vi "ADIS16470 Loop.vi"(8 "error in":errorcluster) -> ()   [LabVIEW 2020]
uses:
  Typedef/ADIS16470 Device Reference.ctl
  Typedef/ADIS16470 Hardware Configuration.ctl
  <vilib>/Rock Robotics/WPI/SPI/WPI_SPIMode.ctl
  <vilib>/Rock Robotics/SystemInterfaces/DIO/FPGA_DIOChannel.ctl
  <vilib>/Rock Robotics/SystemInterfaces/spilib/spi_bus.ctl
  Typedef/ADIS16470 Status.ctl
  Typedef/ADIS16470 Data.ctl
  Typedef/ADIS16470 Process.ctl
  Typedef/ADIS16470 Command Type.ctl
  <vilib>/Rock Robotics/SystemInterfaces/CounterEncoderSourceConvertion/FPGA_CounterEncoderSourceConvertionLVSourceType.ctl
  <vilib>/Rock Robotics/SystemInterfaces/DIO/FPGA_DIODigitalSourceChannel.ctl
  <vilib>/Rock Robotics/SystemInterfaces/AnalogTrigger/FPGA_AnalogTriggerIndex.ctl
  <vilib>/Rock Robotics/SystemInterfaces/AnalogTrigger/FPGA_AnalogTriggerOutType.ctl
  <vilib>/Rock Robotics/WPI/SPI/WPI_SPIDevRef.ctl
  Typedef/ADIS16470 Register.ctl
  <vilib>/Rock Robotics/WPI/Counter/WPI_CounterDigitalInputToDigitalSource.vi
panel:
  out "Offset Bias":i16[](array[numeric])
  in  "ADIS16470DevRef":T1={"DevStatus"={"status"=FALSE, "code"=0, "source"=""}, "Hardware Config"={"SPI Clock Rate (Hz)"=1000000.0, "IMU SPI Mode (3)"=enum."Mode 3 (Clk Idle High,Sample on Trailing)", "IMU Reset Pin"=enum."SPI Port CS2", "IMU SPI Bus"=enum."SPI On-Board, CS0", "IMU Data Ready Pin"=enum."SPI Port CS1", "Stall Config"={"Pow2BytesPerRead"=255, "StallTicks"=640, "CsToSclkTicks"=5}}, "Calibration Complete"=refnum, "Status Reference"=refnum, "Position Reference"=refnum, "Velocity Reference"=refnum, "Sychronous Process VI"=refnum, "Cmd FIFO"=refnum, "Source"={"DevStatus"={"status"=FALSE, "code"=0, "source"=""}, "AnalogTriggerMode?"=FALSE, "DigitalMode"={"DIO Channel"=enum."Disabled"}, "AnalogTriggerMode"={"AnalogTriggerIndex"=enum."Trig 0", "OutputType"=enum."InWindow"}}, "Data FIFO"=refnum, "Calibration Time (ms)"=5}
  in  "Main Name":string
  # "XG_BIAS_LOW"
  # "XG_BIAS_HIGH"
  # "YG_BIAS_LOW"
  # "YG_BIAS_HIGH"
  # "ZG_BIAS_LOW"
  # "ZG_BIAS_HIGH"
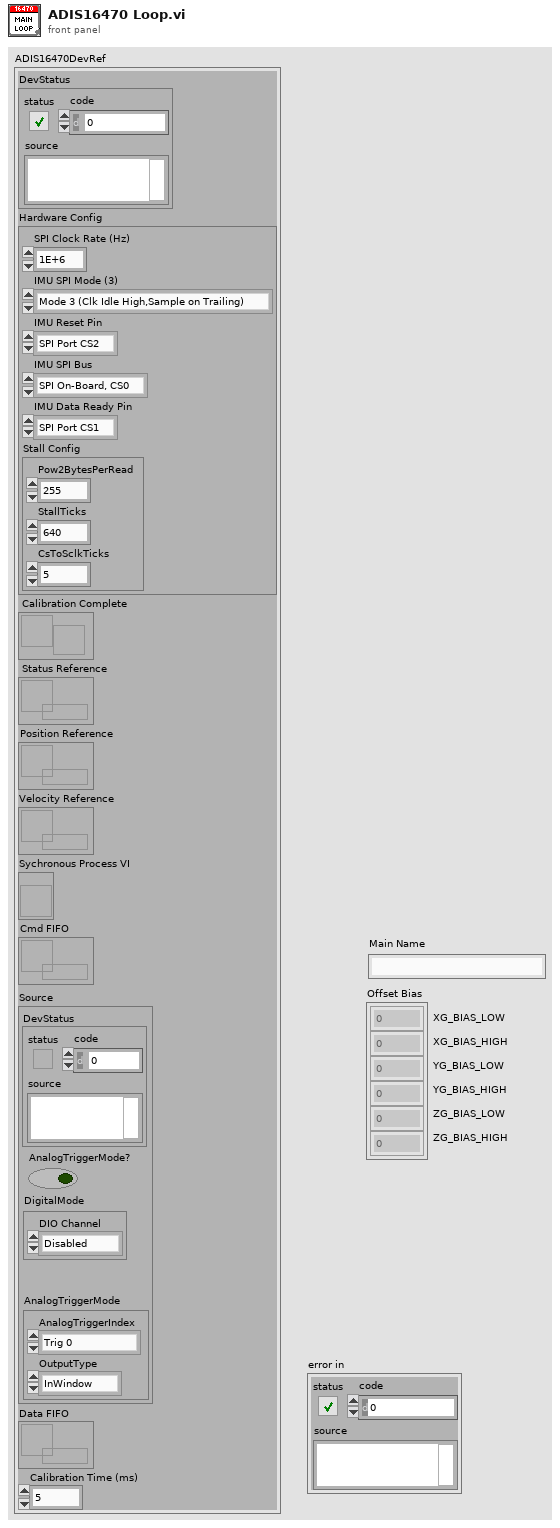
[diagram p1: front panel]
types:
  T1 = typedef "ADIS16470 Device Reference.ctl" = cluster{"DevStatus":errorcluster, "Hardware Config":T2, "Calibration Complete":refnum<notifier>, "Status Reference":refnum<data-value>, "Position Reference":refnum<data-value>, "Velocity Reference":refnum<data-value>, "Sychronous Process VI":T6, "Cmd FIFO":refnum<k33>, "Source":T7, "Data FIFO":refnum<k33>, "Calibration Time (ms)":u32}
  T2 = typedef "ADIS16470 Hardware Configuration.ctl" = cluster{"SPI Clock Rate (Hz)":dbl, "IMU SPI Mode (3)":T3, "IMU Reset Pin":T4, "IMU SPI Bus":T5, "IMU Data Ready Pin":T4, "Stall Config":cluster{"Pow2BytesPerRead":u8, "StallTicks":u16, "CsToSclkTicks":u8}}
  T3 = typedef "WPI_SPIMode.ctl" = enum16{"Mode 0 (Clk Idle Low,Sample on Leading)", "Mode 1 (Clk Idle Low,Sample on Trailing)", "Mode 2 (Clk Idle High,Sample on Leading)", "Mode 3 (Clk Idle High,Sample on Trailing)"}
  T4 = typedef "FPGA_DIOChannel.ctl" = enum8{"DIO 0", "DIO 1", "DIO 2", "DIO 3", "DIO 4", "DIO 5", "DIO 6", "DIO 7", "DIO 8", "DIO 9", "DIO MXP 0", "DIO MXP 1", "DIO MXP 2", "DIO MXP 3", "DIO MXP 4", "DIO MXP 5", "DIO MXP 6", "DIO MXP 7", "DIO MXP 8", "DIO MXP 9", "DIO MXP 10", "DIO MXP 11", "DIO MXP 12", "DIO MXP 13", "DIO MXP 14", "DIO MXP 15", "SPI Port CS1", "SPI Port CS2", "SPI Port CS3", "SPI Port MISO", "SPI Port MOSI", "Invalid"}
  T5 = typedef "spi_bus.ctl" = enum16{"SPI On-Board, CS0", "SPI On-Board, CS1", "SPI On-Board, CS2", "SPI On-Board, CS3", "SPI MXP", "Invalid"}
  T6 = typedef "ADIS16470 Process.ctl" = refnum<vi>
  T7 = typedef "FPGA_CounterEncoderSourceConvertionLVSourceType.ctl" = cluster{"DevStatus":errorcluster, "AnalogTriggerMode?":bool, "DigitalMode":cluster{"DIO Channel":T8}, "AnalogTriggerMode":cluster{"AnalogTriggerIndex":T9, "OutputType":T10}}
  T8 = typedef "FPGA_DIODigitalSourceChannel.ctl" = enum8{"DIO 0", "DIO 1", "DIO 2", "DIO 3", "DIO 4", "DIO 5", "DIO 6", "DIO 7", "DIO 8", "DIO 9", "DIO MXP 0", "DIO MXP 1", "DIO MXP 2", "DIO MXP 3", "DIO MXP 4", "DIO MXP 5", "DIO MXP 6", "DIO MXP 7", "DIO MXP 8", "DIO MXP 9", "DIO MXP 10", "DIO MXP 11", "DIO MXP 12", "DIO MXP 13", "DIO MXP 14", "DIO MXP 15", "SPI Port CS1", "SPI Port CS2", "SPI Port CS3", "SPI Port MISO", "SPI Port MOSI", "Disabled"}
  T9 = typedef "FPGA_AnalogTriggerIndex.ctl" = enum8{"Trig 0", "Trig 1", "Trig 2", "Trig 3", "Trig 4", "Trig 5", "Trig 6", "Trig 7", "Invalid"}
  T10 = typedef "FPGA_AnalogTriggerOutType.ctl" = enum16{"InWindow", "TriggerState", "Rising", "Falling"}
  T11 = typedef "WPI_SPIDevRef.ctl" = cluster{"DevStatus":errorcluster, "Handle":i32, "SPI Bus":T5}
  T12 = typedef "ADIS16470 Data.ctl" = cluster{"XAngle":dbl, "YAngle":dbl, "ZAngle":dbl}
  T13 = typedef "ADIS16470 Register.ctl" = u8
  T14 = cluster{"SPIDevRef":T11, "Data Counter":u16, "Reset":bool, "Digital Source":T7, "Bytes Per Sample":u32, "Position":T12, "Velocity":T12, "ADIS16470DevRef":T1, "TimeStampPrev":u32, "Sensor to Robot Rotation":dbl[][], "Data Packet":T13[], "AutoSPI Active?":bool, "Delay Factor":dbl}
  T15 = typedef "ADIS16470 Status.ctl" = cluster{"Calibrated?":bool, "IMU Detected?":bool}
  T16 = typedef "ADIS16470 Command Type.ctl" = cluster{"Command":enum16{"None", "Reset", "Recalibrate"}, "Data":u32}
  T17 = typedef "WPI_DigitalOutputDevRef.ctl" = cluster{"DIO Channel":T4, "DevStatus":errorcluster}
  T18 = typedef "WPI_DigitalInputDevRef.ctl" = cluster{"DevStatus":errorcluster, "DIO Channel":T4}
  T19 = cluster{"Pow2BytesPerRead":u8, "StallTicks":u16, "CsToSclkTicks":u8}
  T20 = enum32{"Bad", "Idle", "Run top level", "Running"}
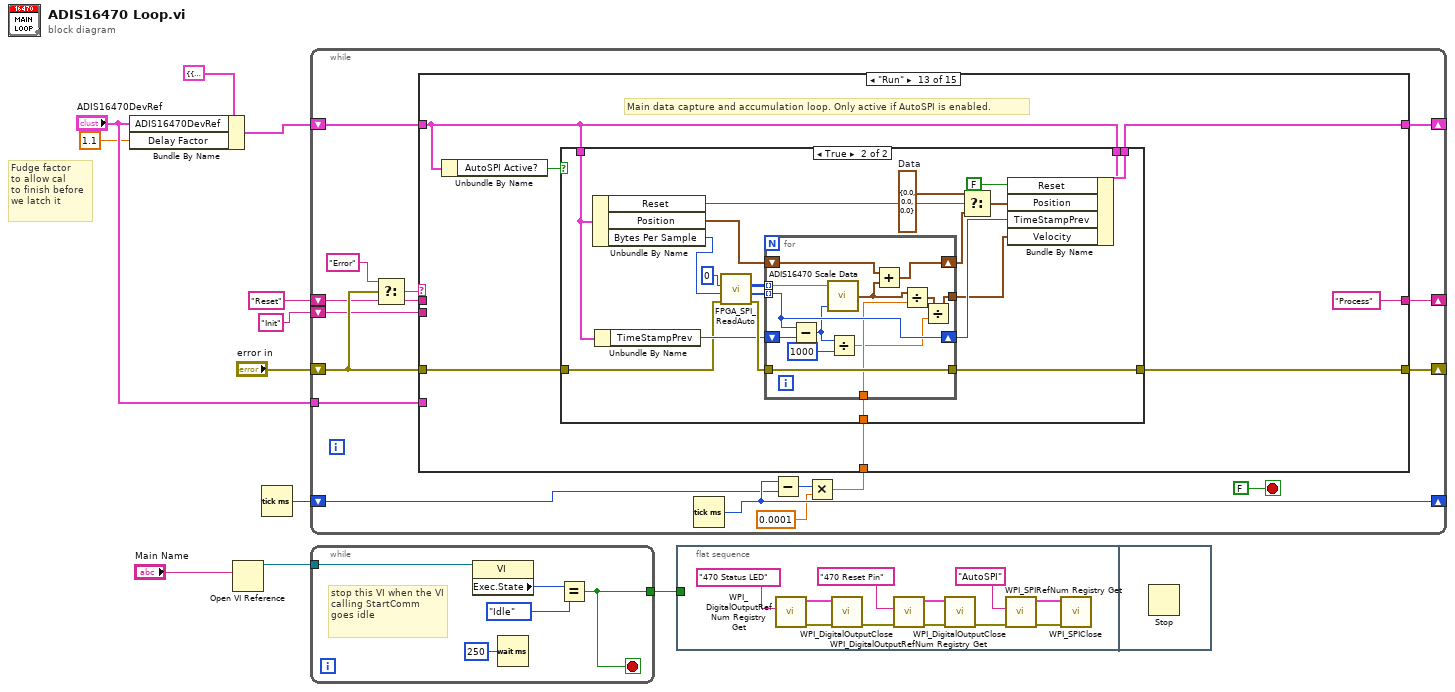
[diagram p0: block diagram]
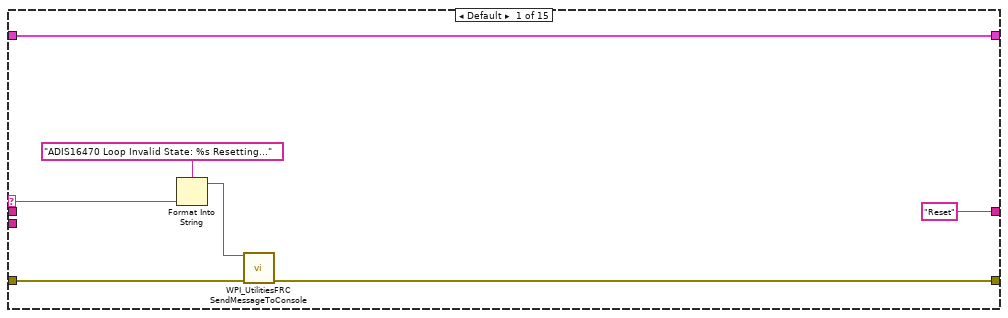
[diagram p2: hidden frame]
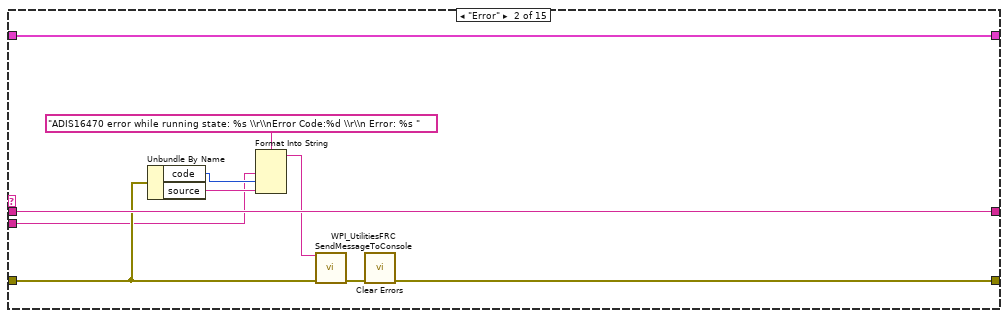
[diagram p3: hidden frame]
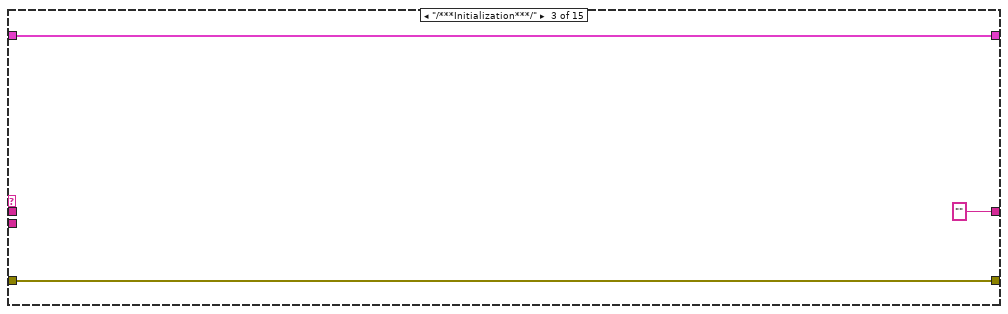
[diagram p4: hidden frame]
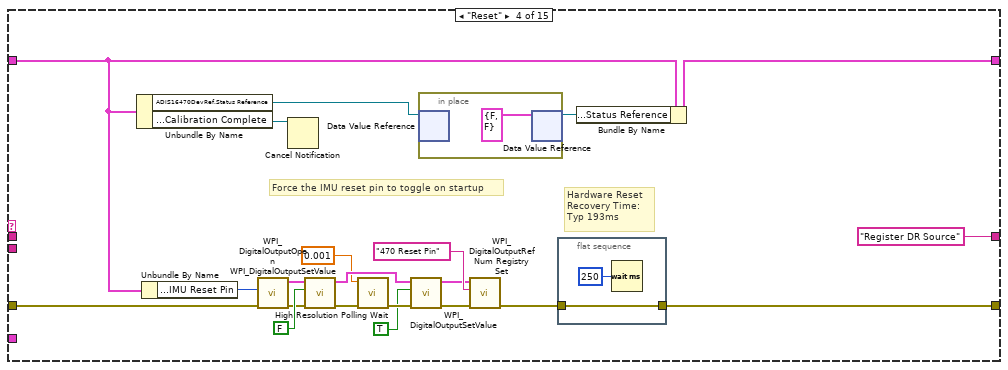
[diagram p5: hidden frame]
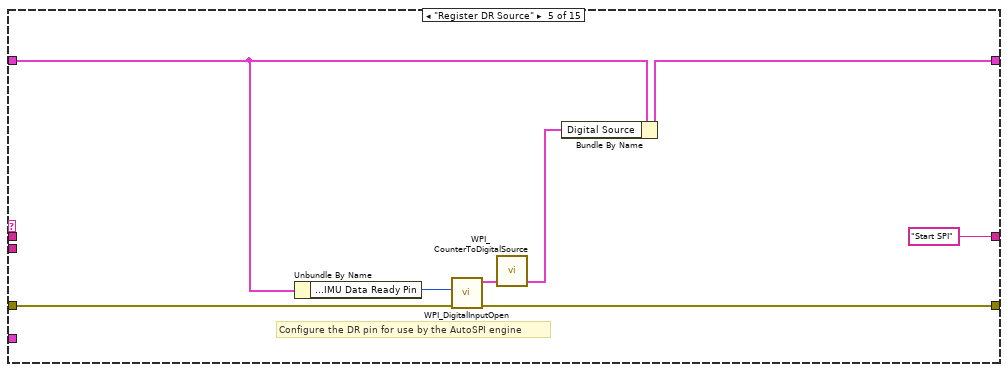
[diagram p6: hidden frame]
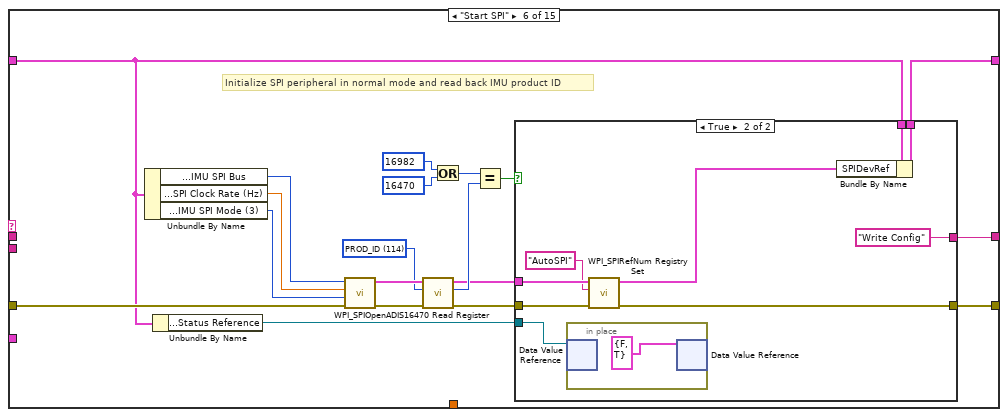
[diagram p7: hidden frame]
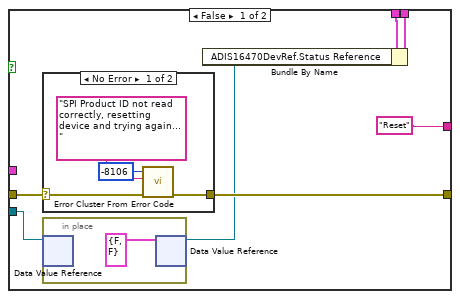
[diagram p8: hidden frame]
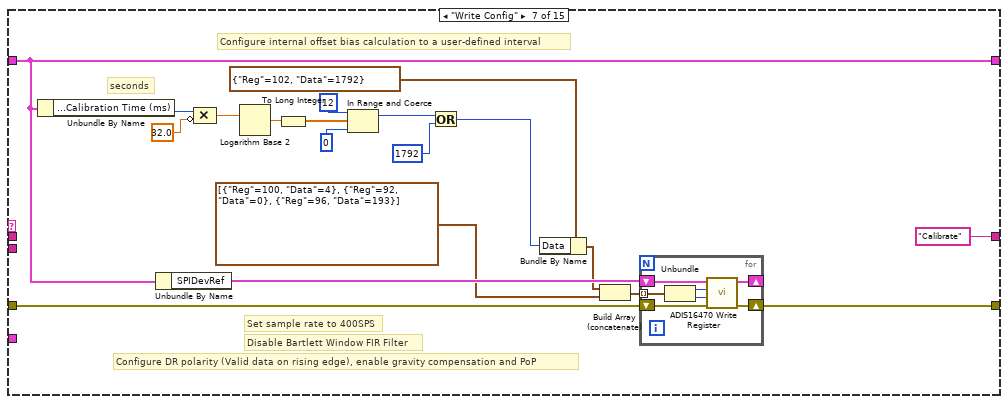
[diagram p10: hidden frame]
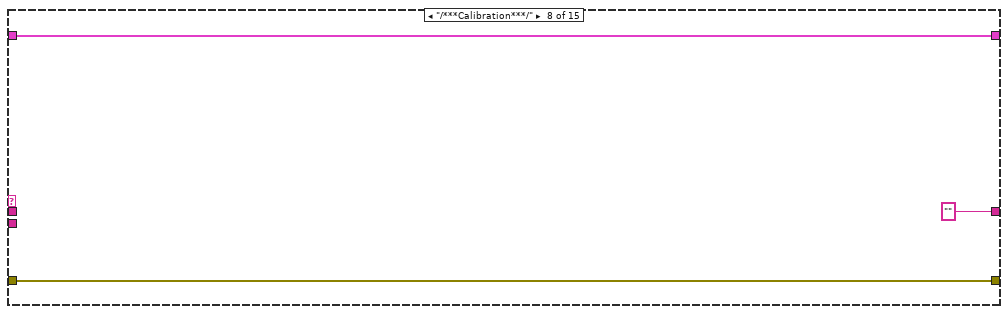
[diagram p11: hidden frame]
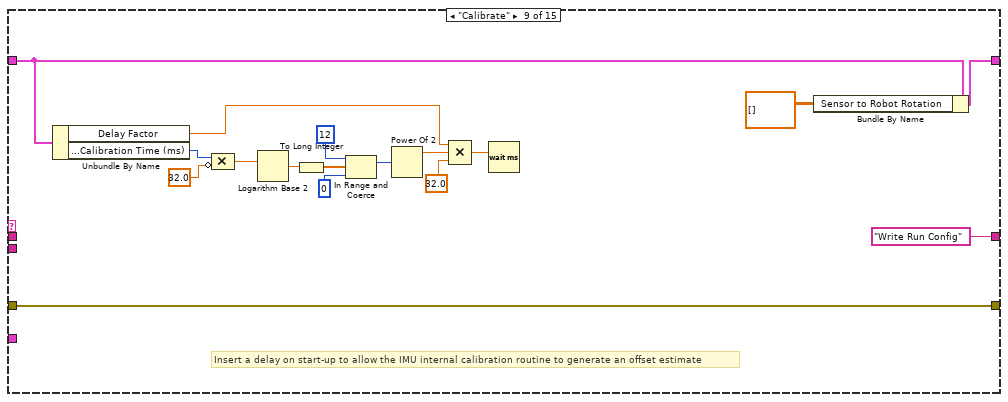
[diagram p12: hidden frame]
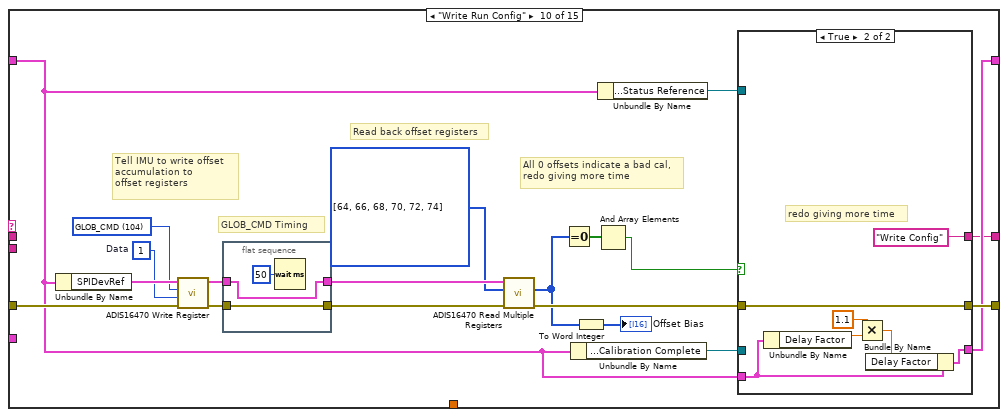
[diagram p13: hidden frame]
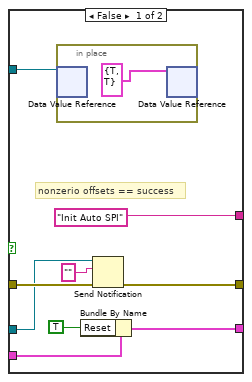
[diagram p14: hidden frame]
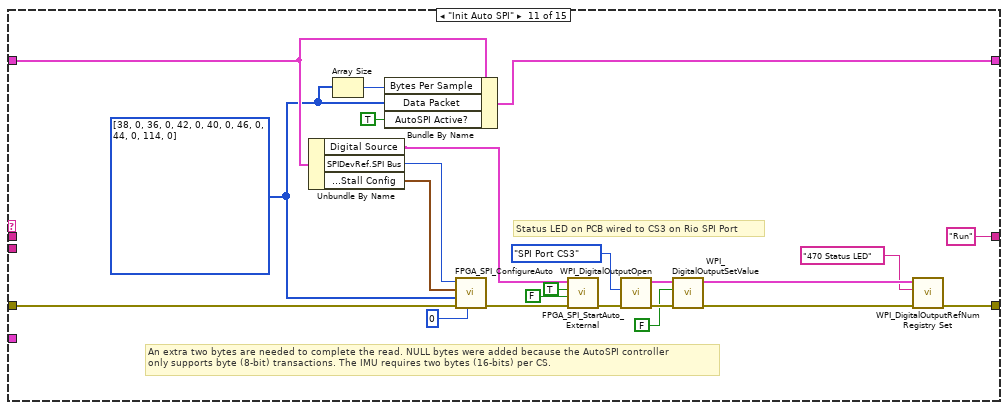
[diagram p15: hidden frame]
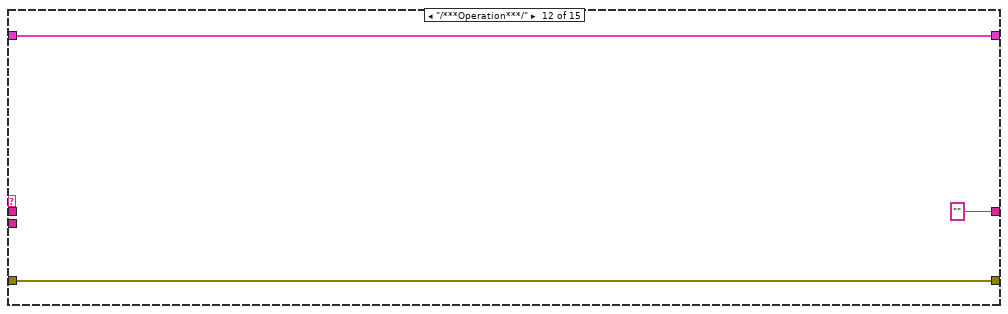
[diagram p16: hidden frame]
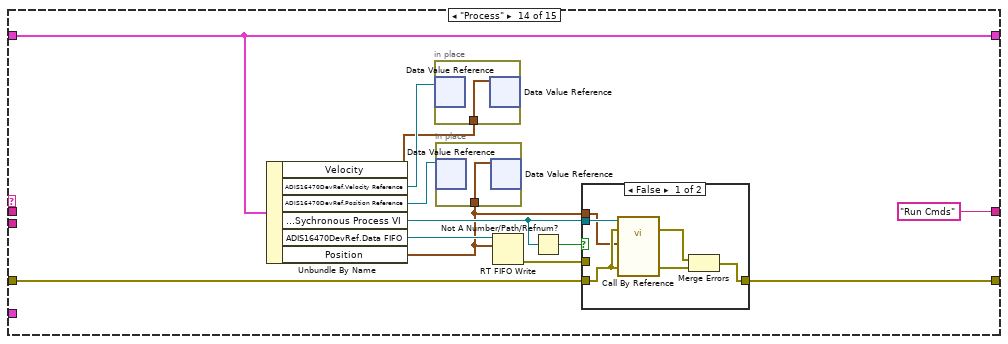
[diagram p18: hidden frame]
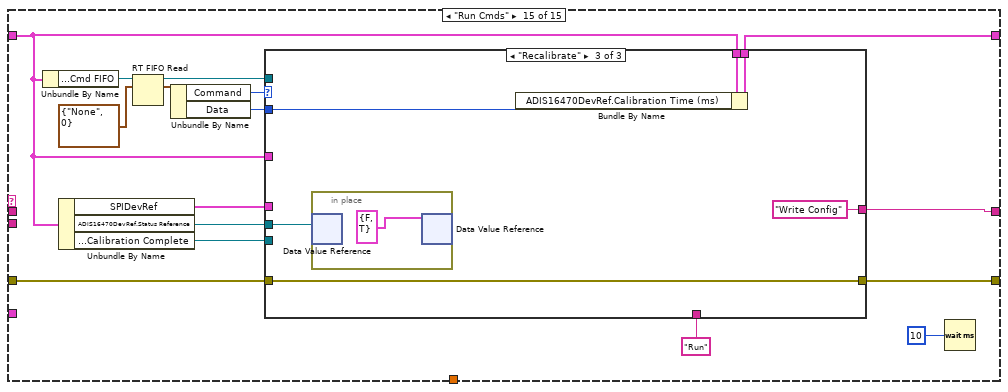
[diagram p20: hidden frame]
diagram:
  # "Fudge factor\nto allow cal\nto finish before\nwe latch it"
  n1 = Bundle By Name(cluster=T14 {"SPIDevRef"={"DevStatus"={"status"=FALSE, "code"=0, "source"=""}, "Handle"=0, "SPI Bus"=enum."SPI On-Board, CS0"}, "Data Counter"=0, "Reset"=FALSE, "Digital Source"={"DevStatus"={"status"=FALSE, "code"=0, "source"=""}, "AnalogTriggerMode?"=FALSE, "DigitalMode"={"DIO Channel"=enum."DIO 1"}, "AnalogTriggerMode"={"AnalogTriggerIndex"=enum."Trig 0", "OutputType"=enum."InWindow"}}, "Bytes Per Sample"=0, "Position"={"XAngle"=0.0, "YAngle"=0.0, "ZAngle"=0.0}, "Velocity"={"XAngle"=0.0, "YAngle"=0.0, "ZAngle"=0.0}, "ADIS16470DevRef"={"DevStatus"={"status"=FALSE, "code"=0, "source"=""}, "Hardware Config"={"SPI Clock Rate (Hz)"=1000000.0, "IMU SPI Mode (3)"=enum."Mode 3 (Clk Idle High,Sample on Trailing)", "IMU Reset Pin"=enum."SPI Port CS2", "IMU SPI Bus"=enum."SPI On-Board, CS0", "IMU Data Ready Pin"=enum."SPI Port CS1", "Stall Config"={"Pow2BytesPerRead"=255, "StallTicks"=640, "CsToSclkTicks"=5}}, "Calibration Complete"=refnum, "Status Reference"=refnum, "Position Reference"=refnum, "Velocity Reference"=refnum, "Sychronous Process VI"=refnum, "Cmd FIFO"=refnum, "Source"={"DevStatus"={"status"=FALSE, "code"=0, "source"=""}, "AnalogTriggerMode?"=FALSE, "DigitalMode"={"DIO Channel"=enum."Disabled"}, "AnalogTriggerMode"={"AnalogTriggerIndex"=enum."Trig 0", "OutputType"=enum."InWindow"}}, "Data FIFO"=refnum, "Calibration Time (ms)"=5}, "TimeStampPrev"=0, "Sensor to Robot Rotation"=[], "Data Packet"=[38, 0, 36, 0, 42, 0, 40, 0, 46, 0, 44, 0, 114, 0], "AutoSPI Active?"=TRUE, "Delay Factor"=1.1} ("Cluster"), "ADIS16470DevRef"="ADIS16470DevRef", "Delay Factor"=1.1) -> (w8:T14)
  n2 = Open VI Reference(vi path="Main Name") -> (vi reference=w10:refnum<vi>)  [unwired: 3 in, 3 out]
  n3 = Tick Count (ms)() -> (millisecond timer value=w1:u32)
  n4 = while {
    shift-right: [w23] -> _
    shift-left: "Reset" -> [w20]
    shift-right: [w25] -> _
    shift-left: w8 -> [w26]
    shift-right: [w24] -> _
    shift-left: "error in" -> [w22]
    shift-left: "Init" -> [w18]
    tunnel: "ADIS16470DevRef" -> [w17]
    shift-right: [w16] -> _
    shift-left: w1 -> [w15]
    stop <- FALSE stop-if-true
    n5 = Select(t="Error", s=w22, f=w20) -> (s? t:f=w21:string)
    n6 = Tick Count (ms)() -> (millisecond timer value=w16:u32)
    n7 = Subtract(x=w16, y=w15) -> (x-y=w14:u32)
    n8 = Multiply(x=w14, y=0.0001) -> (x*y=w12:dbl)
    n9 = case shown="\"Run\"" w21 {
      selector: w21 -> [w33 _ _ _ _ _ _ _ _ _ _ _ _ _ _]
      tunnel: w26 -> [w34 w44 w47 w51 w75 w81 w130 w150 w163 w170 w222 w233 w236 w286 w301]
      tunnel: [w34 w44 w47 w50 w78 w89 w130 w150 w166 w171 w221 w233 w239 w286 w308] -> w25
      tunnel: w22 -> [w32 w40 w46 w66 w77 w95 w138 w149 w165 w186 w229 w232 w238 w284 w310]
      tunnel: [w31 w41 w46 w64 w72 w88 w137 w149 w165 w177 w213 w232 w237 w283 w309] -> w24
      tunnel: ["Reset" w43 "" "Register DR Source" "Start SPI" w90 "Calibrate" "" "Write Run Config" w169 "Run" "" "Process" "Run Cmds" w298] -> w23
      tunnel: w20 -> [_ w43 _ _ _ _ _ _ _ _ _ _ _ _ _]
      tunnel: w18 -> [_ w35 _ _ _ _ _ _ _ _ _ _ _ _ _]
      tunnel: w17 -> [_ _ _ _ _ _ _ _ _ _ _ _ _ _ _]
      tunnel: w12 -> [_ _ _ _ _ _ _ _ _ _ _ _ w234 _ _]
      frame Default {
        n10 = Format Into String(format string="ADIS16470 Loop Invalid State: %s Resetting...", w33) -> (resulting string=w30:string)  [unwired: 2 in, 1 out]
        n11 = call <vilib>:"WPI_UtilitiesFRC SendMessageToConsole.vi"("Message"=w30, "error in (no error)"=w32) -> ("error out"=w31:errorcluster)  [unwired: 13 in]
      }
      frame "Error" {
        n12 = Unbundle By Name(w40) -> ("code"=w37:i32, "source"=w36:string)
        n13 = Format Into String(format string="ADIS16470 error while running state: %s \\r\\nError Code:%d \\r\\n Error: %s ", w35, w37, w36) -> (resulting string=w39:string)  [unwired: 2 in, 1 out]
        n14 = call <vilib>:"WPI_UtilitiesFRC SendMessageToConsole.vi"("Message"=w39, "error in (no error)"=w40) -> ("error out"=w42:errorcluster)  [unwired: 13 in]
        n15 = call <vilib>:"Clear Errors.vi"("error in (no error)"=w42) -> ("error out"=w41:errorcluster)  [unwired: 5 in, 1 out]
      }
      frame "/***Initialization***/" {
      }
      frame "Reset" {
        # "Hardware Reset Recovery Time: Typ 193ms"
        # "Force the IMU reset pin to toggle on startup"
        n16 = Unbundle By Name(w51) -> ("ADIS16470DevRef.Status Reference"=w49:refnum<data-value>, "ADIS16470DevRef.Calibration Complete"=w63:refnum<notifier>)
        n17 = Unbundle By Name(w51) -> ("ADIS16470DevRef.Hardware Config.IMU Reset Pin"=w67:T4)
        n18 = call <vilib>:"WPI_DigitalOutputOpen.vi"("error in (no error)"=w66, "DIO Channel"=w67) -> ("error out"=w61:errorcluster, "DigitalOutputDevRef"=w68:T17)  [unwired: 8 in]
        n19 = Cancel Notification(0:w63) -> ()  [unwired: 1 in, 3 out]
        n20 = call <vilib>:"WPI_DigitalOutputSetValue.vi"("error in (no error)"=w61, "Value"=FALSE, "DigitalOutputDevRef"=w68) -> ("error out"=w58:errorcluster, "DigitalOutputDevRef"=w56:T17)  [unwired: 7 in]
        n21 = call <vilib>:"High Resolution Polling Wait.vi"("error in (no error)"=w58, "seconds to wait"=0.001) -> ("error out"=w57:errorcluster)  [unwired: 9 in]
        n22 = call <vilib>:"WPI_DigitalOutputSetValue.vi"("error in (no error)"=w57, "Value"=TRUE, "DigitalOutputDevRef"=w56) -> ("error out"=w53:errorcluster, "DigitalOutputDevRef"=w54:T17)  [unwired: 7 in]
        n23 = in-place {
          n24 = in-place-dvr #1(w49) -> ()  [unwired: 2 out]
          n25 = in-place-dvr #1(T15 {"Calibrated?"=FALSE, "IMU Detected?"=FALSE} ("element")) -> (w48:refnum<data-value>)  [unwired: 1 out]
        }
        n26 = call <vilib>:"WPI_DigitalOutputRefNum Registry Set.vi"("error in (no error)"=w53, "refnum name"="470 Reset Pin", "DigitalOutputDevRef"=w54) -> ("error out"=w59:errorcluster)  [unwired: 7 in, 1 out]
        n27 = flat-sequence {
          tunnel: [w71] -> w64
          tunnel: w59 -> [w71]
          frame #0 {
            n28 = Wait (ms)(milliseconds to wait=u32 250) -> ()  [unwired: 1 out]
          }
        }
        n29 = Bundle By Name(cluster=w51, "ADIS16470DevRef.Status Reference"=w48) -> (w50:T14)
      }
      frame "Register DR Source" {
        # "Configure the DR pin for use by the AutoSPI engine"
        n30 = Unbundle By Name(w75) -> ("ADIS16470DevRef.Hardware Config.IMU Data Ready Pin"=w74:T4)
        n31 = call <vilib>:"WPI_DigitalInputOpen.vi"("error in (no error)"=w77, "DIO Channel"=w74) -> ("error out"=w72:errorcluster, "DigitalInputDevRef"=w76:T18)  [unwired: 8 in]
        n32 = call-poly <vilib>:"WPI_CounterToDigitalSource.vi"("DigitalInputDevRef"=w76) -> ("Digital Source"=w73:T7)  [unwired: 6 in]
        n33 = Bundle By Name(cluster=w75, "Digital Source"=w73) -> (w78:T14)
      }
      frame "Start SPI" {
        w83 = T13 114 items=["Reserved1"=0, "DIAG_STAT"=2, "X_GYRO_LOW"=4, "X_GYRO_OUT"=6, "Y_GYRO_LOW"=8, "Y_GYRO_OUT"=10, "Z_GYRO_LOW"=12, "Z_GYRO_OUT"=14, "X_ACCL_LOW"=16, "X_ACCL_OUT"=18, "Y_ACCL_LOW"=20, "Y_ACCL_OUT"=22, "Z_ACCL_LOW"=24, "Z_ACCL_OUT"=26, "TEMP_OUT"=28, "TIME_STAMP"=30, "Reseved2"=32, "DATA_CNTR"=34, "X_DELTANG_LOW"=36, "X_DELTANG_OUT"=38, "Y_DELTANG_LOW"=40, "Y_DELTANG_OUT"=42, "Z_DELTANG_LOW"=44, "Z_DELTANG_OUT"=46, "X_DELTVEL_LOW"=48, "X_DELTVEL_OUT"=50, "Y_DELTVEL_LOW"=52, "Y_DELTVEL_OUT"=54, "Z_DELTVEL_LOW"=56, "Z_DELTVEL_OUT"=58, "Reserved3"=60, "Reserved4"=62, "XG_BIAS_LOW"=64, "XG_BIAS_HIGH"=66, "YG_BIAS_LOW"=68, "YG_BIAS_OUT"=70, "ZG_BIAS_LOW"=72, "ZG_BIAS_OUT"=74, "XA_BIAS_LOW"=76, "XA_BIAS_HIGH"=78, "YA_BIAS_LOW"=80, "YA_BIAS_OUT"=82, "ZA_BIAS_LOW"=84, "ZA_BIAS_OUT"=86, "Reserved5"=88, "Reserved6"=90, "FILT_CTRL"=92, "Reserved5"=94, "MSC_CTRL"=96, "UP_SCALE"=98, "DEC_RATE"=100, "NULL_CNFG"=102, "GLOB_CMD"=104, "Reserved6"=106, "FIRM_REV"=108, "FIRM_DM"=110, "FIRM_Y"=112, "PROD_ID"=114, "SERIAL_NUM"=116, "USER_SCR1"=118, "USER_SCR2"=120, "USER_SCR3"=122, "FLSHCNT_LOW"=124, "FLSHCNT_HIGH"=126] ("ADIS16448 Register")
        # "Initialize SPI peripheral in normal mode and read back IMU product ID"
        n34 = Unbundle By Name(w81) -> ("ADIS16470DevRef.Hardware Config.IMU SPI Bus"=w91:T5, "ADIS16470DevRef.Hardware Config.SPI Clock Rate (Hz)"=w92:dbl, "ADIS16470DevRef.Hardware Config.IMU SPI Mode (3)"=w93:T3)
        n35 = Unbundle By Name(w81) -> ("ADIS16470DevRef.Status Reference"=w80:refnum<data-value>)
        n36 = call <vilib>:"WPI_SPIOpen.vi"("error in"=w95, "Mode (3)"=w93, "Clock Rate (Hz)"=w92, "SPI Bus"=w91) -> ("error out"=w85:errorcluster, "SPIDevRef"=w84:T11)  [unwired: 6 in]
        n37 = call "ADIS16470 Read Register.vi"("error in (no error)"=w85, "ADIS16470 Register"=w83, "SPIDevRef in"=w84) -> ("error out"=w86:errorcluster, "Register Value"=w87:u16, "SPIDevRef out"=w82:T11)  [unwired: 6 in]
        n38 = Or(x=u16 16982 ("y"), y=u16 16470) -> (x .or. y?=w96:u16)
        n39 = Equal?(x=w96, y=w87) -> (x = y?=w94:bool)
        n40 = case shown="True" w94 {
          tunnel: ["Reset" "Write Config"] -> w90
          tunnel: w81 -> [w101 w119]
          tunnel: [w100 w118] -> w89
          tunnel: [w104 w114] -> w88
          tunnel: w86 -> [w103 w117]
          tunnel: w82 -> [_ w116]
          tunnel: w80 -> [w102 w112]
          frame False {
            n41 = case shown="No Error" w103 {
              selector: w103 -> [w109 w111]
              tunnel: [w110 w111] -> w104
              frame No Error {
                n42 = call <vilib>:"Error Cluster From Error Code.vi"("error in (no error)"=w109, "error message (\"\")"="SPI Product ID not read correctly, resetting device and trying again..." ("error message (\"\")"), "error code (0)"=-8106) -> ("error out"=w110:errorcluster)  [unwired: 6 in]
              }
              frame Error {
              }
            }
            n43 = in-place {
              n44 = in-place-dvr #2(w102) -> ()  [unwired: 2 out]
              n45 = in-place-dvr #2(T15 {"Calibrated?"=FALSE, "IMU Detected?"=FALSE} ("element")) -> (w99:refnum<data-value>)  [unwired: 1 out]
            }
            n46 = Bundle By Name(cluster=w101, "ADIS16470DevRef.Status Reference"=w99) -> (w100:T14)
          }
          frame True {
            n47 = in-place {
              n48 = in-place-dvr #3(w112) -> ()  [unwired: 2 out]
              n49 = in-place-dvr #3(T15 {"Calibrated?"=FALSE, "IMU Detected?"=TRUE} ("element")) -> ()  [unwired: 2 out]
            }
            n50 = call <vilib>:"WPI_SPIRefNum Registry Set.vi"("error in (no error)"=w117, "refnum name"="AutoSPI", "SPIDevRef"=w116) -> ("error out"=w114:errorcluster, "SPIDevRef"=w115:T11)  [unwired: 7 in]
            n51 = Bundle By Name(cluster=w119, "SPIDevRef"=w115) -> (w118:T14)
          }
        }
      }
      frame "Write Config" {
        # "seconds"
        # "Set sample rate to 400SPS"
        # "Configure internal offset bias calculation to a user-defined interval"
        # "Configure DR polarity (Valid data on rising edge), enable gravity compensation and PoP"
        # "Disable Bartlett Window FIR Filter"
        n52 = Unbundle By Name(w130) -> ("ADIS16470DevRef.Calibration Time (ms)"=w125:u32)
        n53 = Unbundle By Name(w130) -> ("SPIDevRef"=w139:T11)
        n54 = Compound Arithmetic op=MULTIPLY(w125, invert 32.0 ("x")) -> (w123:dbl)
        n55 = Logarithm Base 2(1:w123) -> (0:w129:dbl)
        n56 = To Long Integer(number=w129) -> (32bit integer=w126:i32)
        n57 = In Range and Coerce(upper limit=12 ("x"), x=w126, lower limit=0 ("x")) -> (coerced(x)=w122:i32)  [unwired: 1 out]
        n58 = Or(x=w122, y=1792 ("Data")) -> (x .or. y?=w131:i32)
        n59 = Bundle By Name(cluster=cluster{"Reg":T13, "Data":i32} {"Reg"=102, "Data"=1792}, "Data"=w131) -> (w133:cluster{"Reg":T13, "Data":i32})
        n60 = Build Array (concatenate)(w133, cluster{"Reg":T13, "Data":u16}[] [{"Reg"=100, "Data"=4}, {"Reg"=92, "Data"=0}, {"Reg"=96, "Data"=193}]) -> (w134:cluster{"Reg":T13, "Data":i32}[])
        n61 = for {
          tunnel: w134 -> [w147] mode=indexing
          shift-right: [w143] -> w137
          shift-left: w138 -> [w142]
          shift-right: [w141] -> _
          shift-left: w139 -> [w144]
          n62 = Unbundle(w147) -> ("Reg"=w146:T13, "Data"=w145:i32)
          n63 = call "ADIS16470 Write Register.vi"("error in (no error)"=w142, "Data"=w145, "Register"=w146, "SPIDevRef in"=w144) -> ("error out"=w143:errorcluster, "SPIDevRef out"=w141:T11)  [unwired: 6 in]
        }
      }
      frame "/***Calibration***/" {
      }
      frame "Calibrate" {
        # "Insert a delay on start-up to allow the IMU internal calibration routine to generate an offset estimate"
        n64 = Unbundle By Name(w163) -> ("Delay Factor"=w151:dbl, "ADIS16470DevRef.Calibration Time (ms)"=w157:u32)
        n65 = Compound Arithmetic op=MULTIPLY(w157, invert 32.0 ("x")) -> (w158:dbl)
        n66 = Logarithm Base 2(1:w158) -> (0:w162:dbl)
        n67 = To Long Integer(number=w162) -> (32bit integer=w160:i32)
        n68 = In Range and Coerce(upper limit=12 ("x"), x=w160, lower limit=0 ("x")) -> (coerced(x)=w155:i32)  [unwired: 1 out]
        n69 = Power Of 2(x=w155) -> (2^x=w154:dbl)
        n70 = Compound Arithmetic op=MULTIPLY(w151, w154, 32.0 ("x")) -> (w152:dbl)
        n71 = Wait (ms)(milliseconds to wait=w152) -> ()  [unwired: 1 out]
        n72 = Bundle By Name(cluster=w163, "Sensor to Robot Rotation"=dbl[][] []) -> (w166:T14)
      }
      frame "Write Run Config" {
        w176 = T13 104 items=["Reserved1"=0, "DIAG_STAT"=2, "X_GYRO_LOW"=4, "X_GYRO_OUT"=6, "Y_GYRO_LOW"=8, "Y_GYRO_OUT"=10, "Z_GYRO_LOW"=12, "Z_GYRO_OUT"=14, "X_ACCL_LOW"=16, "X_ACCL_OUT"=18, "Y_ACCL_LOW"=20, "Y_ACCL_OUT"=22, "Z_ACCL_LOW"=24, "Z_ACCL_OUT"=26, "TEMP_OUT"=28, "TIME_STAMP"=30, "Reseved2"=32, "DATA_CNTR"=34, "X_DELTANG_LOW"=36, "X_DELTANG_OUT"=38, "Y_DELTANG_LOW"=40, "Y_DELTANG_OUT"=42, "Z_DELTANG_LOW"=44, "Z_DELTANG_OUT"=46, "X_DELTVEL_LOW"=48, "X_DELTVEL_OUT"=50, "Y_DELTVEL_LOW"=52, "Y_DELTVEL_OUT"=54, "Z_DELTVEL_LOW"=56, "Z_DELTVEL_OUT"=58, "Reserved3"=60, "Reserved4"=62, "XG_BIAS_LOW"=64, "XG_BIAS_HIGH"=66, "YG_BIAS_LOW"=68, "YG_BIAS_OUT"=70, "ZG_BIAS_LOW"=72, "ZG_BIAS_OUT"=74, "XA_BIAS_LOW"=76, "XA_BIAS_HIGH"=78, "YA_BIAS_LOW"=80, "YA_BIAS_OUT"=82, "ZA_BIAS_LOW"=84, "ZA_BIAS_OUT"=86, "Reserved5"=88, "Reserved6"=90, "FILT_CTRL"=92, "Reserved5"=94, "MSC_CTRL"=96, "UP_SCALE"=98, "DEC_RATE"=100, "NULL_CNFG"=102, "GLOB_CMD"=104, "Reserved6"=106, "FIRM_REV"=108, "FIRM_DM"=110, "FIRM_Y"=112, "PROD_ID"=114, "SERIAL_NUM"=116, "USER_SCR1"=118, "USER_SCR2"=120, "USER_SCR3"=122, "FLSHCNT_LOW"=124, "FLSHCNT_HIGH"=126] ("Register")
        w185 = u16 1  # Data
        w181 = T13[] [64, 66, 68, 70, 72, 74] items=["Reserved1"=0, "DIAG_STAT"=2, "X_GYRO_LOW"=4, "X_GYRO_OUT"=6, "Y_GYRO_LOW"=8, "Y_GYRO_OUT"=10, "Z_GYRO_LOW"=12, "Z_GYRO_OUT"=14, "X_ACCL_LOW"=16, "X_ACCL_OUT"=18, "Y_ACCL_LOW"=20, "Y_ACCL_OUT"=22, "Z_ACCL_LOW"=24, "Z_ACCL_OUT"=26, "TEMP_OUT"=28, "TIME_STAMP"=30, "Reseved2"=32, "DATA_CNTR"=34, "X_DELTANG_LOW"=36, "X_DELTANG_OUT"=38, "Y_DELTANG_LOW"=40, "Y_DELTANG_OUT"=42, "Z_DELTANG_LOW"=44, "Z_DELTANG_OUT"=46, "X_DELTVEL_LOW"=48, "X_DELTVEL_OUT"=50, "Y_DELTVEL_LOW"=52, "Y_DELTVEL_OUT"=54, "Z_DELTVEL_LOW"=56, "Z_DELTVEL_OUT"=58, "Reserved3"=60, "Reserved4"=62, "XG_BIAS_LOW"=64, "XG_BIAS_HIGH"=66, "YG_BIAS_LOW"=68, "YG_BIAS_HIGH"=70, "ZG_BIAS_LOW"=72, "ZG_BIAS_HIGH"=74, "XA_BIAS_LOW"=76, "XA_BIAS_HIGH"=78, "YA_BIAS_LOW"=80, "YA_BIAS_HIGH"=82, "ZA_BIAS_LOW"=84, "ZA_BIAS_HIGH"=86, "Reserved5"=88, "Reserved6"=90, "FILT_CTRL"=92, "Reserved5"=94, "MSC_CTRL"=96, "UP_SCALE"=98, "DEC_RATE"=100, "NULL_CNFG"=102, "GLOB_CMD"=104, "Reserved6"=106, "FIRM_REV"=108, "FIRM_DM"=110, "FIRM_Y"=112, "PROD_ID"=114, "SERIAL_NUM"=116, "USER_SCR1"=118, "USER_SCR2"=120, "USER_SCR3"=122, "FLSHCNT_LOW"=124, "FLSHCNT_HIGH"=126] ("Registers")
        # "All 0 offsets indicate a bad cal,\nredo giving more time"
        # "Tell IMU to write offset \naccumulation to \noffset registers"
        # "GLOB_CMD Timing"
        # "Read back offset registers"
        n73 = Unbundle By Name(w170) -> ("SPIDevRef"=w187:T11)
        n74 = call "ADIS16470 Write Register.vi"("error in (no error)"=w186, "Data"=w185, "Register"=w176, "SPIDevRef in"=w187) -> ("error out"=w184:errorcluster, "SPIDevRef out"=w183:T11)  [unwired: 6 in]
        n75 = flat-sequence {
          tunnel: w184 -> [w207]
          tunnel: [w207] -> w175
          tunnel: w183 -> [w205]
          tunnel: [w205] -> w182
          frame #0 {
            n76 = Wait (ms)(milliseconds to wait=u32 50) -> ()  [unwired: 1 out]
          }
        }
        n77 = call "ADIS16470 Read Multiple Registers.vi"("error in (no error)"=w175, "Registers"=w181, "SPIDevRefIn"=w182) -> ("error out"=w179:errorcluster, "Values"=w174:u16[])  [unwired: 6 in, 1 out]
        n78 = Equal To 0?(x=w174) -> (x = 0?=w173:bool[])
        n79 = Unbundle By Name(w170) -> ("ADIS16470DevRef.Calibration Complete"=w178:refnum<notifier>)
        n80 = To Word Integer(number=w174) -> (16bit integer=→"Offset Bias":i16[])
        n81 = Unbundle By Name(w170) -> ("ADIS16470DevRef.Status Reference"=w168:refnum<data-value>)
        n82 = And Array Elements(Boolean array=w173) -> (logical AND=w172:bool)
        n83 = case shown="True" w172 {
          tunnel: w179 -> [w196 w204]
          tunnel: w178 -> [w195 _]
          tunnel: [w194 w204] -> w177
          tunnel: w170 -> [w191 w202]
          tunnel: [w190 w203] -> w171
          tunnel: ["Init Auto SPI" "Write Config"] -> w169
          tunnel: w168 -> [w188 _]
          frame False {
            # "nonzerio offsets == success"
            n84 = in-place {
              n85 = in-place-dvr #4(w188) -> ()  [unwired: 2 out]
              n86 = in-place-dvr #4(T15 {"Calibrated?"=TRUE, "IMU Detected?"=TRUE} ("element")) -> ()  [unwired: 2 out]
            }
            n87 = Bundle By Name(cluster=w191, "Reset"=TRUE ("First Run")) -> (w190:T14)
            n88 = Send Notification(notification="", notifier=w195, error in (no error)=w196) -> (error out=w194:errorcluster)  [unwired: 1 out]
          }
          frame True {
            # "redo giving more time"
            n89 = Unbundle By Name(w202) -> ("Delay Factor"=w201:dbl)
            n90 = Multiply(x=1.1, y=w201) -> (x*y=w199:dbl)
            n91 = Bundle By Name(cluster=w202, "Delay Factor"=w199) -> (w203:T14)
          }
        }
      }
      frame "Init Auto SPI" {
        w208 = T13[] [38, 0, 36, 0, 42, 0, 40, 0, 46, 0, 44, 0, 114, 0] items=["NULL"=0, "DIAG_STAT"=2, "X_GYRO_LOW"=4, "X_GYRO_OUT"=6, "Y_GYRO_LOW"=8, "Y_GYRO_OUT"=10, "Z_GYRO_LOW"=12, "Z_GYRO_OUT"=14, "X_ACCL_LOW"=16, "X_ACCL_OUT"=18, "Y_ACCL_LOW"=20, "Y_ACCL_OUT"=22, "Z_ACCL_LOW"=24, "Z_ACCL_OUT"=26, "TEMP_OUT"=28, "TIME_STAMP"=30, "Reseved2"=32, "DATA_CNTR"=34, "X_DELTANG_LOW"=36, "X_DELTANG_OUT"=38, "Y_DELTANG_LOW"=40, "Y_DELTANG_OUT"=42, "Z_DELTANG_LOW"=44, "Z_DELTANG_OUT"=46, "X_DELTVEL_LOW"=48, "X_DELTVEL_OUT"=50, "Y_DELTVEL_LOW"=52, "Y_DELTVEL_OUT"=54, "Z_DELTVEL_LOW"=56, "Z_DELTVEL_OUT"=58, "Reserved3"=60, "Reserved4"=62, "XG_BIAS_LOW"=64, "XG_BIAS_HIGH"=66, "YG_BIAS_LOW"=68, "YG_BIAS_HIGH"=70, "ZG_BIAS_LOW"=72, "ZG_BIAS_HIGH"=74, "XA_BIAS_LOW"=76, "XA_BIAS_HIGH"=78, "YA_BIAS_LOW"=80, "YA_BIAS_HIGH"=82, "ZA_BIAS_LOW"=84, "ZA_BIAS_HIGH"=86, "Reserved5"=88, "Reserved6"=90, "FILT_CTRL"=92, "Reserved5"=94, "MSC_CTRL"=96, "UP_SCALE"=98, "DEC_RATE"=100, "NULL_CNFG"=102, "GLOB_CMD"=104, "Reserved6"=106, "FIRM_REV"=108, "FIRM_DM"=110, "FIRM_Y"=112, "PROD_ID"=114, "SERIAL_NUM"=116, "USER_SCR1"=118, "USER_SCR2"=120, "USER_SCR3"=122, "FLSHCNT_LOW"=124, "FLSHCNT_HIGH"=126] ("Registers")
        # "Status LED on PCB wired to CS3 on Rio SPI Port"
        # "An extra two bytes are needed to complete the read. NULL bytes were added because the AutoSPI controller \nonly supports byte (8-bit) transactions. The IMU requires two bytes (16-bits) per CS."
        n92 = Unbundle By Name(w222) -> ("Digital Source"=w210:T7, "SPIDevRef.SPI Bus"=w209:T5, "ADIS16470DevRef.Hardware Config.Stall Config"=w212:T19)
        n93 = Array Size(array=w208) -> (size(s)=w220:i32)
        n94 = Bundle By Name(cluster=w222, "Bytes Per Sample"=w220, "Data Packet"=w208, "AutoSPI Active?"=TRUE) -> (w221:T14)
        n95 = call <vilib>:"FPGA_SPI_ConfigureAuto.vi"("SPI Auto Zero Byte Count"=u8 0, "error in"=w229, "SPI Auto TX Byte Array"=w208, "Stall Config"=w212, "SPI Bus"=w209) -> ("error out"=w227:errorcluster)  [unwired: 6 in]
        n96 = call <vilib>:"FPGA_SPI_StartAuto_External.vi"("error in (no error)"=w227, "Falling Edge"=FALSE, "Rising Edge"=TRUE, "Source"=w210) -> ("error out"=w223:errorcluster)  [unwired: 7 in]
        n97 = call <vilib>:"WPI_DigitalOutputOpen.vi"("error in (no error)"=w223, "DIO Channel"=FPGA_DIOChannel."SPI Port CS3") -> ("error out"=w219:errorcluster, "DigitalOutputDevRef"=w218:T17)  [unwired: 8 in]
        n98 = call <vilib>:"WPI_DigitalOutputSetValue.vi"("error in (no error)"=w219, "Value"=FALSE, "DigitalOutputDevRef"=w218) -> ("error out"=w216:errorcluster, "DigitalOutputDevRef"=w215:T17)  [unwired: 7 in]
        n99 = call <vilib>:"WPI_DigitalOutputRefNum Registry Set.vi"("error in (no error)"=w216, "refnum name"="470 Status LED", "DigitalOutputDevRef"=w215) -> ("error out"=w213:errorcluster)  [unwired: 7 in, 1 out]
      }
      frame "/***Operation***/" {
      }
      frame "Run" {
        # "Main data capture and accumulation loop. Only active if AutoSPI is enabled."
        n100 = Unbundle By Name(w236) -> ("AutoSPI Active?"=w235:bool)
        n101 = case shown="True" w235 {
          tunnel: [w242 w262] -> w239
          tunnel: w238 -> [w241 w247]
          tunnel: [w241 w252] -> w237
          tunnel: w236 -> [w242 w251]
          tunnel: w236 -> [_ w248]
          tunnel: w234 -> [_ w243]
          frame False {
          }
          frame True {
            w246 = T12 {"XAngle"=0.0, "YAngle"=0.0, "ZAngle"=0.0}  # Data
            n102 = Unbundle By Name(w248) -> ("Reset"=w260:bool, "Position"=w255:T12, "Bytes Per Sample"=w259:u32)
            n103 = Unbundle By Name(w248) -> ("TimeStampPrev"=w250:u32)
            n104 = call <vilib>:"FPGA_SPI_ReadAuto.vi"("error in (no error)"=w247, "Bytes per Sample"=w259, "Samples to Read"=u32 0) -> ("error out"=w253:errorcluster, "Timestamps"=w256:u32[], "Data"=w257:u8[][])  [unwired: 6 in]
            n105 = for {
              tunnel: w257 -> [w271] mode=indexing
              tunnel: w256 -> [w273] mode=indexing
              shift-right: [w270] -> w254
              shift-left: w255 -> [w275]
              tunnel: w253 -> [w272]
              tunnel: [w272] -> w252
              shift-right: [w273] -> w249
              shift-left: w250 -> [w274]
              tunnel: [w263] -> w244
              tunnel: w243 -> [w268]
              n106 = Subtract(x=w273, y=w274) -> (x-y=w267:u32)
              n107 = call "ADIS16470 Scale Data.vi"("TimeStamp"=w267, "Data In"=w271) -> ("Data"=w269:T12)  [unwired: 3 in]
              n108 = Divide(x=w267, y=u32 1000) -> (x/y=w265:dbl)
              n109 = Add(x=w275, y=w269) -> (x+y=w270:T12)
              n110 = Divide(x=w269, y=w268) -> (x/y=w264:T12)
              n111 = Divide(x=w264, y=w265) -> (x/y=w263:T12)
            }
            n112 = Select(t=w246, s=w260, f=w254) -> (s? t:f=w245:T12)
            n113 = Bundle By Name(cluster=w251, "Reset"=FALSE ("First Run"), "Position"=w245, "TimeStampPrev"=w249, "Velocity"=w244) -> (w262:T14)
          }
        }
      }
      frame "Process" {
        n114 = Unbundle By Name(w286) -> ("Velocity"=w276:T12, "ADIS16470DevRef.Velocity Reference"=w277:refnum<data-value>, "ADIS16470DevRef.Position Reference"=w280:refnum<data-value>, "ADIS16470DevRef.Sychronous Process VI"=w281:T6, "ADIS16470DevRef.Data FIFO"=w285:refnum<k33>, "Position"=w278:T12)
        n115 = in-place {
          in-place-border: w276 -> [w288]
          n116 = in-place-dvr #5(w277) -> ()  [unwired: 2 out]
          n117 = in-place-dvr #5(w288) -> ()  [unwired: 2 out]
        }
        n118 = in-place {
          in-place-border: w278 -> [w289]
          n119 = in-place-dvr #6(w280) -> ()  [unwired: 2 out]
          n120 = in-place-dvr #6(w289) -> ()  [unwired: 2 out]
        }
        n121 = RT FIFO Write(0:w285, 1:w278) -> (11:w279:errorcluster)  [unwired: 3 in, 3 out]
        n122 = Not A Number/Path/Refnum?(number/path/refnum=w281) -> (NaN/Path/Refnum?=w282:bool)
        n123 = case shown="False" w282 {
          tunnel: w284 -> [w291 w296]
          tunnel: [w295 w296] -> w283
          tunnel: w281 -> [w294 _]
          tunnel: w279 -> [_ _]
          tunnel: w278 -> [w290 _]
          frame False {
            n124 = call-by-ref "?"(reference=w294, error in=w291, 8:"error in (no error)"=w291, "element"=w290) -> (error out=w292:errorcluster, 0:"error out"=w293:errorcluster)  [unwired: 9 in, 1 out]
            n125 = Merge Errors(w292, w293) -> (w295:errorcluster)
          }
          frame True {
          }
        }
      }
      frame "Run Cmds" {
        n126 = Unbundle By Name(w301) -> ("ADIS16470DevRef.Cmd FIFO"=w311:refnum<k33>)
        n127 = Unbundle By Name(w301) -> ("SPIDevRef"=w300:T11, "ADIS16470DevRef.Status Reference"=w306:refnum<data-value>, "ADIS16470DevRef.Calibration Complete"=w307:refnum<notifier>)
        n128 = RT FIFO Read(0:w311, 1:T16 {"Command"=enum."None", "Data"=0} ("element")) -> (8:w305:refnum<k33>, 9:w304:T16)  [unwired: 2 in, 3 out]
        n129 = Unbundle By Name(w304) -> ("Command"=w303:enum16{"None", "Reset", "Recalibrate"}, "Data"=w302:u32)
        n130 = case shown="\"Recalibrate\"" w303 {
          tunnel: w301 -> [w314 w320 w323]
          tunnel: w310 -> [w315 w319 w325]
          tunnel: [w315 w319 w325] -> w309
          tunnel: [w314 w318 w324] -> w308
          tunnel: w307 -> [_ _ _]
          tunnel: w306 -> [_ _ w321]
          tunnel: w305 -> [_ _ _]
          tunnel: w302 -> [_ _ w322]
          tunnel: w301 -> [_ _ _]
          tunnel: w300 -> [_ _ _]
          tunnel: [w313 "Run" "Write Config"] -> w298
          tunnel: "Run" -> [w313 _ _]
          frame "None", Default {
          }
          frame "Reset" {
            n131 = Bundle By Name(cluster=w320, "Reset"=TRUE ("First Run")) -> (w318:T14)
          }
          frame "Recalibrate" {
            n132 = in-place {
              n133 = in-place-dvr #7(w321) -> ()  [unwired: 2 out]
              n134 = in-place-dvr #7(T15 {"Calibrated?"=FALSE, "IMU Detected?"=TRUE} ("element")) -> ()  [unwired: 2 out]
            }
            n135 = Bundle By Name(cluster=w323, "ADIS16470DevRef.Calibration Time (ms)"=w322) -> (w324:T14)
          }
        }
        n136 = Wait (ms)(milliseconds to wait=u32 10) -> ()  [unwired: 1 out]
      }
    }
  }
  n137 = while {
    tunnel: w10 -> [w329]
    tunnel: [w328] -> w5
    stop <- w328 stop-if-true
    # "stop this VI when the VI calling StartComm goes idle"
    n138 = property class="VI"(reference=w329) -> ("Exec.State"=w331:T20)  [unwired: 1 in, 2 out]
    n139 = Wait (ms)(milliseconds to wait=u32 250) -> ()  [unwired: 1 out]
    n140 = Equal?(x=w331, y=T20."Idle" ("Execution:State")) -> (x = y?=w328:bool)
  }
  n141 = flat-sequence {
    tunnel: w5 -> [_]
    frame #0 {
      n142 = call <vilib>:"WPI_DigitalOutputRefNum Registry Get.vi"("refnum name"="470 Status LED") -> ("error out"=w342:errorcluster, "DigitalOutputDevRef"=w341:T17)  [unwired: 9 in]
      n143 = call <vilib>:"WPI_DigitalOutputClose.vi"("error in (no error)"=w342, "DigitalOutputDevRef"=w341) -> ("error out"=w340:errorcluster)  [unwired: 9 in]
      n144 = call <vilib>:"WPI_DigitalOutputRefNum Registry Get.vi"("error in (no error)"=w340, "refnum name"="470 Reset Pin") -> ("error out"=w338:errorcluster, "DigitalOutputDevRef"=w337:T17)  [unwired: 8 in]
      n145 = call <vilib>:"WPI_DigitalOutputClose.vi"("error in (no error)"=w338, "DigitalOutputDevRef"=w337) -> ("error out"=w336:errorcluster)  [unwired: 9 in]
      n146 = call <vilib>:"WPI_SPIRefNum Registry Get.vi"("error in (no error)"=w336, "refnum name"="AutoSPI") -> ("error out"=w334:errorcluster, "SPIDevRef"=w333:T11)  [unwired: 8 in]
      n147 = call <vilib>:"WPI_SPIClose.vi"("error in (no error)"=w334, "SPIDevRef"=w333) -> ()  [unwired: 9 in, 1 out]
    }
    frame #1 {
      n148 = Stop() -> ()  [unwired: 1 in]
    }
  }
